vi "奇偶比较器（I8）.vi"(0 "整数":i8) -> (2 "奇数?":bool, 3 "偶数?":bool)   [LabVIEW 2013]
doc: "Check if an integer is odd.\n\nAuthored by David A. Moore\nsupport@mooregoodideas.com\nwww.mooregoodideas.com\n\nCopyright (c) 2010, Moore Good Ideas, Inc.\n\nAll rights reserved.\n\nRedistribution and use in source and binary forms, with or without modification, are permitted provided that the following conditions are met:\n\n * Redistributions of source code must retain the above copyright notice, this list of conditions and the following disclaimer.\n * Redistributions in binary form must reproduce the above copyright notice, this list of conditions and the following disclaimer in the documentation and/or other materials provided with the distribution.\n * Neither the name of Moore Good Ideas, Inc. nor the names of its contributors may be used to endorse or promote products derived from this software without specific prior written permission.\n\nTHIS SOFTWARE IS PROVIDED BY THE COPYRIGHT HOLDERS AND CONTRIBUTORS \"AS IS\" AND ANY EXPRESS OR IMPLIED WARRANTIES, INCLUDING, BUT NOT LIMITED TO, THE IMPLIED WARRANTIES OF MERCHANTABILITY AND FITNESS FOR A PARTICULAR PURPOSE ARE DISCLAIMED. IN NO EVENT SHALL THE COPYRIGHT OWNER OR CONTRIBUTORS BE LIABLE FOR ANY DIRECT, INDIRECT, INCIDENTAL, SPECIAL, EXEMPLARY, OR CONSEQUENTIAL DAMAGES (INCLUDING, BUT NOT LIMITED TO, PROCUREMENT OF SUBSTITUTE GOODS OR SERVICES; LOSS OF USE, DATA, OR PROFITS; OR BUSINESS INTERRUPTION) HOWEVER CAUSED AND ON ANY THEORY OF LIABILITY, WHETHER IN CONTRACT, STRICT LIABILITY, OR TORT (INCLUDING NEGLIGENCE OR OTHERWISE) ARISING IN ANY WAY OUT OF THE USE OF THIS SOFTWARE, EVEN IF ADVISED OF THE POSSIBILITY OF SUCH DAMAGE."
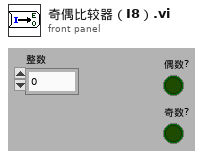
[diagram p1: front panel]
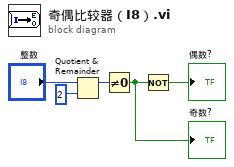
[diagram p0: block diagram]
diagram:
  n1 = Quotient & Remainder(x="整数", y=i8 2) -> (x-y*floor(x/y)=w3:i8)  [unwired: 1 out]
  n2 = Not Equal To 0?(x=w3) -> (x != 0?=w1:bool)
  "奇数?" <- w1
  n3 = Not(x=w1) -> (.not. x?=→"偶数?":bool)
